vi "Release Module Semaphore.vi"(8 "error in":errorcluster) -> (0 "error out":errorcluster)   [LabVIEW 2021, in "Safety.lvlib"]
doc: "Release the module semaphore.\n_____\nBased on DQMH Project Template 7.0.1.1316."
uses:
  Safety.lvlib
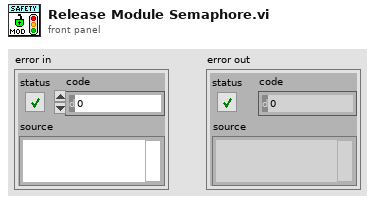
[diagram p1: front panel]
types:
  T1 = typedef "Semaphore RefNum" = refnum<k1>
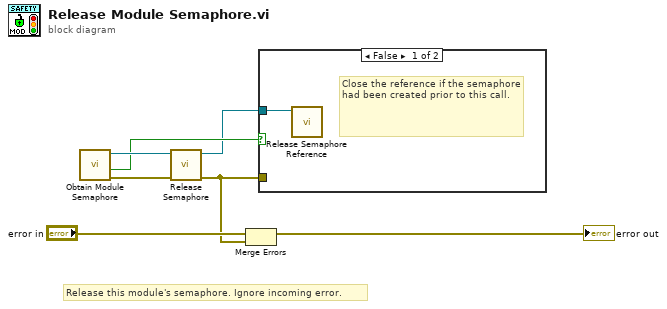
[diagram p0: block diagram]
diagram:
  # "Release this module's semaphore. Ignore incoming error."
  n1 = call "Obtain Module Semaphore.vi"() -> ("error out"=w5:errorcluster, "created new?"=w2:bool, "semaphore"=w3:T1)  [unwired: 9 in]
  n2 = call <vilib>:"Release Semaphore.vi"("error in (no error)"=w5, "semaphore"=w3) -> ("error out"=w4:errorcluster, "semaphore out"=w1:T1)  [unwired: 4 in]
  n3 = Merge Errors("error in", w4) -> (→"error out":errorcluster)
  n4 = case shown="False" w2 {
    tunnel: w4 -> [_ _]
    tunnel: w1 -> [w8 _]
    frame False {
      # "Close the reference if the semaphore had been created prior to this call."
      n5 = call <vilib>:"Release Semaphore Reference.vi"("semaphore"=w8) -> ()  [unwired: 9 in, 2 out]
    }
    frame True {
    }
  }
